vi "请求注销.vi"(8 "error in (no error)":errorcluster caption="错误输入（无错误）", 10 "数据采集.lvclass":refnum<class "数据采集.lvclass">, 11 "数据分析 输入":refnum<class "数据分析.lvclass"> caption="DNL_LabVIEW Object in") -> (0 "error out":errorcluster caption="错误输出", 2 "数据采集.lvclass":refnum<class "数据采集.lvclass">, 3 "数据分析 输出":refnum<class "数据分析.lvclass"> caption="DNL_LabVIEW Object out")   [LabVIEW 2011]
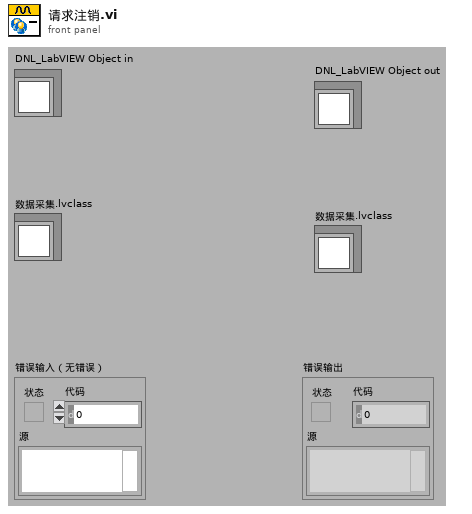
[diagram p1: front panel]
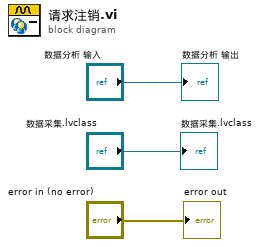
[diagram p0: block diagram]
diagram:
  "error out" <- "error in (no error)"
  "数据分析 输出" <- "数据分析 输入"
  "数据采集.lvclass" <- "数据采集.lvclass"
